vi "Vision Processing.vi"(4 "error in (no error)":errorcluster, 5 "Color Components":T1={"Hue"={110.0, 142.0}, "Sat"={138.0, 255.0}, "Val"={139.0, 198.0}} {"Val" scale=0.0..255.0; "Sat" scale=0.0..255.0; "Hue" scale=0.0..255.0 scale format="%#_3g"}, 6 "Image Size":T2=enum."320x240", 7 "Enable Vision":bool=TRUE) -> (3 "Distances":T4(array[cluster]))   [LabVIEW 2013]
doc: "This VI runs in parallel to other tasks. It gets images from the camera, processes them for color or shape and use that information to affect robot behavior."
uses:
  Vision/TargetType.ctl
  <vilib>/Rock Robotics/WPI/Camera/WPI_CameraImageSize.ctl
panel:
  in  "Annotate":bool
  in  "Score Limit":dbl=70.0
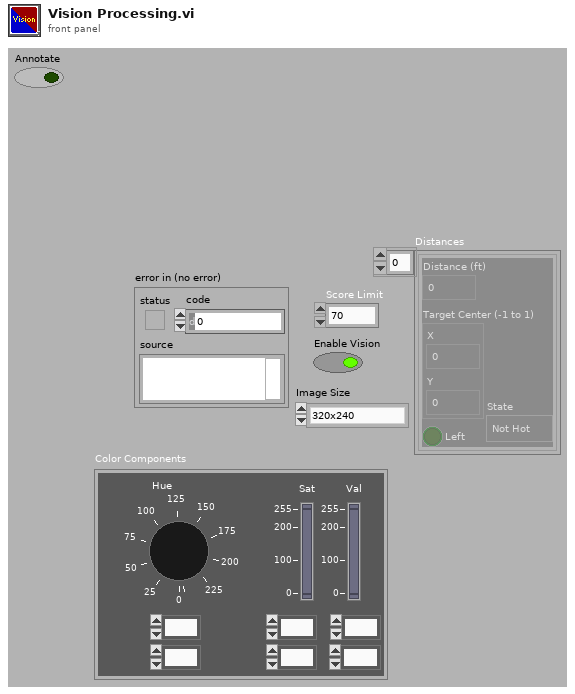
[diagram p1: front panel]
types:
  T1 = cluster{"Hue":cluster{dbl, dbl}, "Sat":cluster{dbl, dbl}, "Val":cluster{dbl, dbl}}
  T2 = typedef "WPI_CameraImageSize.ctl" = enum16{"640x480", "320x240", "160x120"}
  T3 = typedef "TargetType.ctl" = enum16{"Not Hot", "Hot"}
  T4 = cluster{"Distance (ft)":dbl, "Target Center (-1 to 1)":cluster{"X":dbl, "Y":dbl}, "Left":bool, "State":T3}[]
  T5 = typedef "Image Type" = u32
  T6 = typedef "WPI_CameraDevRef.ctl" = cluster{"Camera Address":string, "CameraStatus":errorcluster, "Acquire Image Notifier":refnum<notifier>}
  T7 = typedef "IMAQ Image.ctl" = refnum<image>
  T8 = cluster{"Horizontal":bool, "Aspect Score":dbl, "Rect Score":dbl, cluster{"Left":dbl, "Top":dbl, "Right":dbl, "Bottom":dbl}, "Equiv H":dbl, "Equiv V":dbl}[]
  T9 = cluster{"Scores":cluster{"Total":dbl, "Left":dbl, "Right":dbl, "Ratio":dbl, "Vertical":dbl, "index":i32, "State":T3}, "Verticals":cluster{"Horizontal?":bool, "Aspect Score":dbl, "Rect Score":dbl, cluster{"Left":dbl, "Top":dbl, "Right":dbl, "Bottom":dbl}, "Equiv H":dbl, "Equiv V":dbl}, "Horizontals":cluster{"Horizontal?":bool, "Aspect Score":dbl, "Rect Score":dbl, cluster{"Left":dbl, "Top":dbl, "Right":dbl, "Bottom":dbl}, "Equiv H":dbl, "Equiv V":dbl}, "Validated":bool}[]
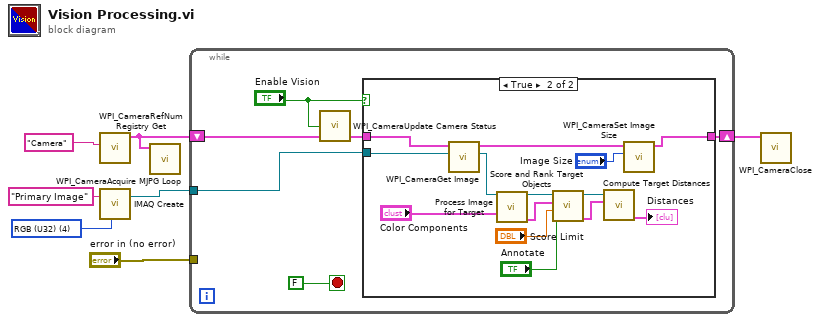
[diagram p0: block diagram]
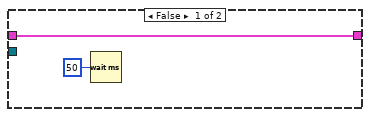
[diagram p2: hidden frame]
diagram:
  w7 = T5 4 items=["Grayscale (U8)", "Grayscale (I16)", "Grayscale (SGL)", "Complex (CSG)", "RGB (U32)", "HSL (U32)", "RGB (U64)"] ("Image Type")
  n1 = call <vilib>:"WPI_CameraRefNum Registry Get.vi"("refnum name"="Camera") -> ("CameraDevRef"=w3:T6)  [unwired: 9 in, 1 out]
  n2 = call "IMAQ Create"("Image Name"="Primary Image", "Image Type"=w7) -> ("New Image"=w5:T7)  [unwired: 2 in, 2 out]
  n3 = call <vilib>:"WPI_CameraAcquire MJPG Loop.vi"("CameraDevRef"=w3) -> ()  [unwired: 11 in]
  n4 = while {
    shift-right: [w12] -> w4
    shift-left: w3 -> [w10]
    tunnel: w5 -> [w11]
    tunnel: "error in (no error)" -> [_]
    stop <- FALSE stop-if-true
    n5 = call <vilib>:"WPI_CameraUpdate Camera Status.vi"("CameraDevRef In"=w10, "Enable Vision"="Enable Vision") -> ("CameraDevRef Out"=w9:T6)  [unwired: 3 in]
    n6 = case shown="True" "Enable Vision" {
      tunnel: w11 -> [_ w28]
      tunnel: [w15 w29] -> w12
      tunnel: w9 -> [w15 w27]
      frame False {
        n7 = Wait (ms)(milliseconds to wait=u32 50) -> ()  [unwired: 1 out]
      }
      frame True {
        n8 = call <vilib>:"WPI_CameraGet Image.vi"("Image"=w28, "CameraDevRef"=w27) -> ("Image Out"=w25:T7, "CameraDevRef Out"=w26:T6)  [unwired: 1 in, 7 out]
        n9 = call "Process Image for Target.vi"("Src Image"=w25, "Color Components"="Color Components") -> ("Src Image Out"=w24:T7, "Particles"=w22:T8)  [unwired: 11 in, 1 out]
        n10 = call "Score and Rank Target Objects.vi"("Annotate"="Annotate", "Score Limit"="Score Limit", "Particles"=w22, "Image in"=w24) -> ("Target Info"=w20:T9, "Annotated Image"=w23:T7)  [unwired: 6 in]
        n11 = call "Compute Target Distances.vi"("Target Info"=w20, "Image in"=w23) -> ("Distances"=→"Distances":T4)  [unwired: 7 in, 2 out]
        n12 = call <vilib>:"WPI_CameraSet Image Size.vi"("Image Size"="Image Size", "CameraDevRef"=w26) -> ("CameraDevRef Out"=w29:T6)  [unwired: 1 in, 8 out]
      }
    }
  }
  n13 = call <vilib>:"WPI_CameraClose.vi"("CameraDevRef"=w4) -> ()  [unwired: 1 in, 10 out]
